vi "PC Streaming Host_2012.vi"() -> ()   [LabVIEW 2012]
uses:
  <vilib>/rvi/interface/nirviOpenFPGA/nirviOpenFPGA.xnode
  <vilib>/rvi/interface/nirviMethod/nirviMethod.xnode
  <vilib>/rvi/errors/niLvFpgaMergeErrorWithErrorCode.vi
  <vilib>/ptbypt/NI_PtbyPt.lvlib
  <vilib>/rvi/interface/nirviCloseFPGA/nirviCloseFPGA.xnode
  <vilib>/rvi/interface/nirviReadWriteControl/nirviReadWriteControl.xnode
  <vilib>/rvi/interface/Simulation/niFpgaSimulationCallBeginRW.vi
  <vilib>/rvi/errors/niLvFpgaAdjustHostInterfaceError.vi
  NiFpgaLv.dll
  <vilib>/Utility/error.llb/Error Cluster From Error Code.vi
  FPGA Bitfiles/TopLevelFPGA1.0.lvbitx
  Program Files/CAEN/HV/CAENHVWrapper/labview/CAENHVWrapper/CAENHVWrapper.lvlib
  <vilib>/FPGAPlugInAG/Dynamic/niLvFpga_ConfigureFifo_Dynamic.vi
  <vilib>/FPGAPlugInAG/Dynamic/niLvFpga_StartFifo_Dynamic.vi
  <vilib>/LabVIEW Targets/FPGA/FlexRIO/CustomFPGAMethods/79XXR_Method_IOModuleStatusImpl.vi
  <vilib>/FPGAPlugInAG/Dynamic/niLvFpga_Run_Dynamic.vi
  <vilib>/FPGAPlugInAG/Dynamic/niLvFpga_ReadFifo_Dynamic.vi
  <vilib>/FPGAPlugInAG/Dynamic/niLvFpga_Close_Dynamic.vi
  <vilib>/FPGAPlugInAG/PXI-7951R/niLvFpga_Open_PXI-7951R.vi
  <vilib>/rvi/interface/common/dynamic/niFpgaDynamicAddResources.vi
  <vilib>/userdefined/High Color/nirio_resource_hc.ctl
panel:
  out "Array":string[][](array[string])
  out "handle HV1":i32
  out "handle HV2":i32
  out "File name":string
  out "Total Data Chunks to Write":dbl
  in  "Tab Control":T1(tab)
  in  "Write mode":bool
  out "directory exists - please wait":u8(slide)
  out "directory ok":bool
  in  "Write Enable":bool=TRUE
  in  "File Path":path=path "C:/Users/admfroukjeg/Documents/test"
  in  "Number of Files to Write":u32=1
  in  "Save 10% of Data?":bool
  out "File Writing Progress (%)":dbl(slide) scale=0.0..100.0
  in  "Location":i16(ring)=1 items=["Purdue", "NIKHEF", "Zurich", "???"]
  in  "PXI address":T2="RIO0" caption="RIO Device"
  in  "Trigger level":i16[](array[numeric])=[4000, 4000, 4000, 4000, 4000, 4000, 4000, 4000] caption="Trigger"
  in  "Channel 0":bool=TRUE caption="Channel 1"
  in  "Channel 1":bool
  in  "Channel 2":bool caption="Channel 1"
  in  "Channel 3":bool caption="Channel 1"
  in  "Channel 4":bool caption="Channel 1"
  in  "Channel 5":bool caption="Channel 1"
  in  "Channel 6":bool caption="Channel 1"
  in  "Channel 7":bool caption="Channel 1"
  in  "Sources":string[](array[combo])
  in  "Serial numbers":string[](array[combo])
  in  "voltage":string[](array[string])=["100", "200", "300", "400", "500", "600", "700", "800"]
  in  "det_type":string[](array[combo])
  out "Voltage HV1":string[][](array[string])
  out "Voltage HV2":string[][](array[string])
  in  "IP adress HV1":string="1_0_0"
  in  "IP adress HV2":string="0_0_0"
  out "handle":i32
  in  "Master Pulser On/Off":bool
  in  "Pulse duration (samples)":u32
  in  "Pulse Separation (samples)":u32
  in  "Testpulse Turnaround Time (samples)":u32=14
  in  "circular buffer length (samples)":u32=1000
  in  "Pretrigger Samples":u32=15
  out "Samples per Data Chunk":u32
  in  "Waveforms per Data Chunk":u32=200 format="%.2p"
  in  "Samples per Waveform":u32=95
  in  "Data Chunks per File":u32=2
  out "Average Throughput":dbl(graph)
  out "Loop Time":u32
  out "Inst. Throughput":dbl format="%#_6p"
  out "Elements in FIFO":u32(graph)
  out "FIFO Overflow":bool
  out "Current Chunk":u32
  out "Current File":i32
  out "Trigger rate":dbl(graph)
  out "Waveform Graph":dynamicdata(graph)
  out "Channel number displayed":i16=-1
  out "XML String":string
  out "error out":errorcluster
  out "UTC format?":bool=TRUE
  out "Stopped":bool
  out "Channel On/Off":bool[](array[boolean])
  in  "stop 2":bool
  in  "stop":bool
  # "Only write every 10th chunk to disk"
  # "Program will stop when number of Files to Write is Complete OR if stop is pressed."
  # "Write continuously"
  # "Write finite number of files"
  # "TODO: Make this look like the \"detectors\" tab"
  # "Waveform/Data Chunk information"
  # "To compare directly on a scope: Horizontal scale: 200 ns/div Vertical scale: ~100 mV/div If 15 pretriggers, delay = 700 ns"
types:
  T1 = enum32{"File", "Detectors", "HV", "Pulser", "DAQ", "Host", "FIFO", "Trigger Rate", "Waveform Display", "XML", "Errors", "Misc."}
  T2 = typedef "nirio_resource_hc.ctl" = tag
  T3 = enum16{"open", "replace", "create", "open or create", "replace or create", "replace or create with confirmation"}
  T4 = enum16{"big-endian, network order", "native, host order", "little-endian"}
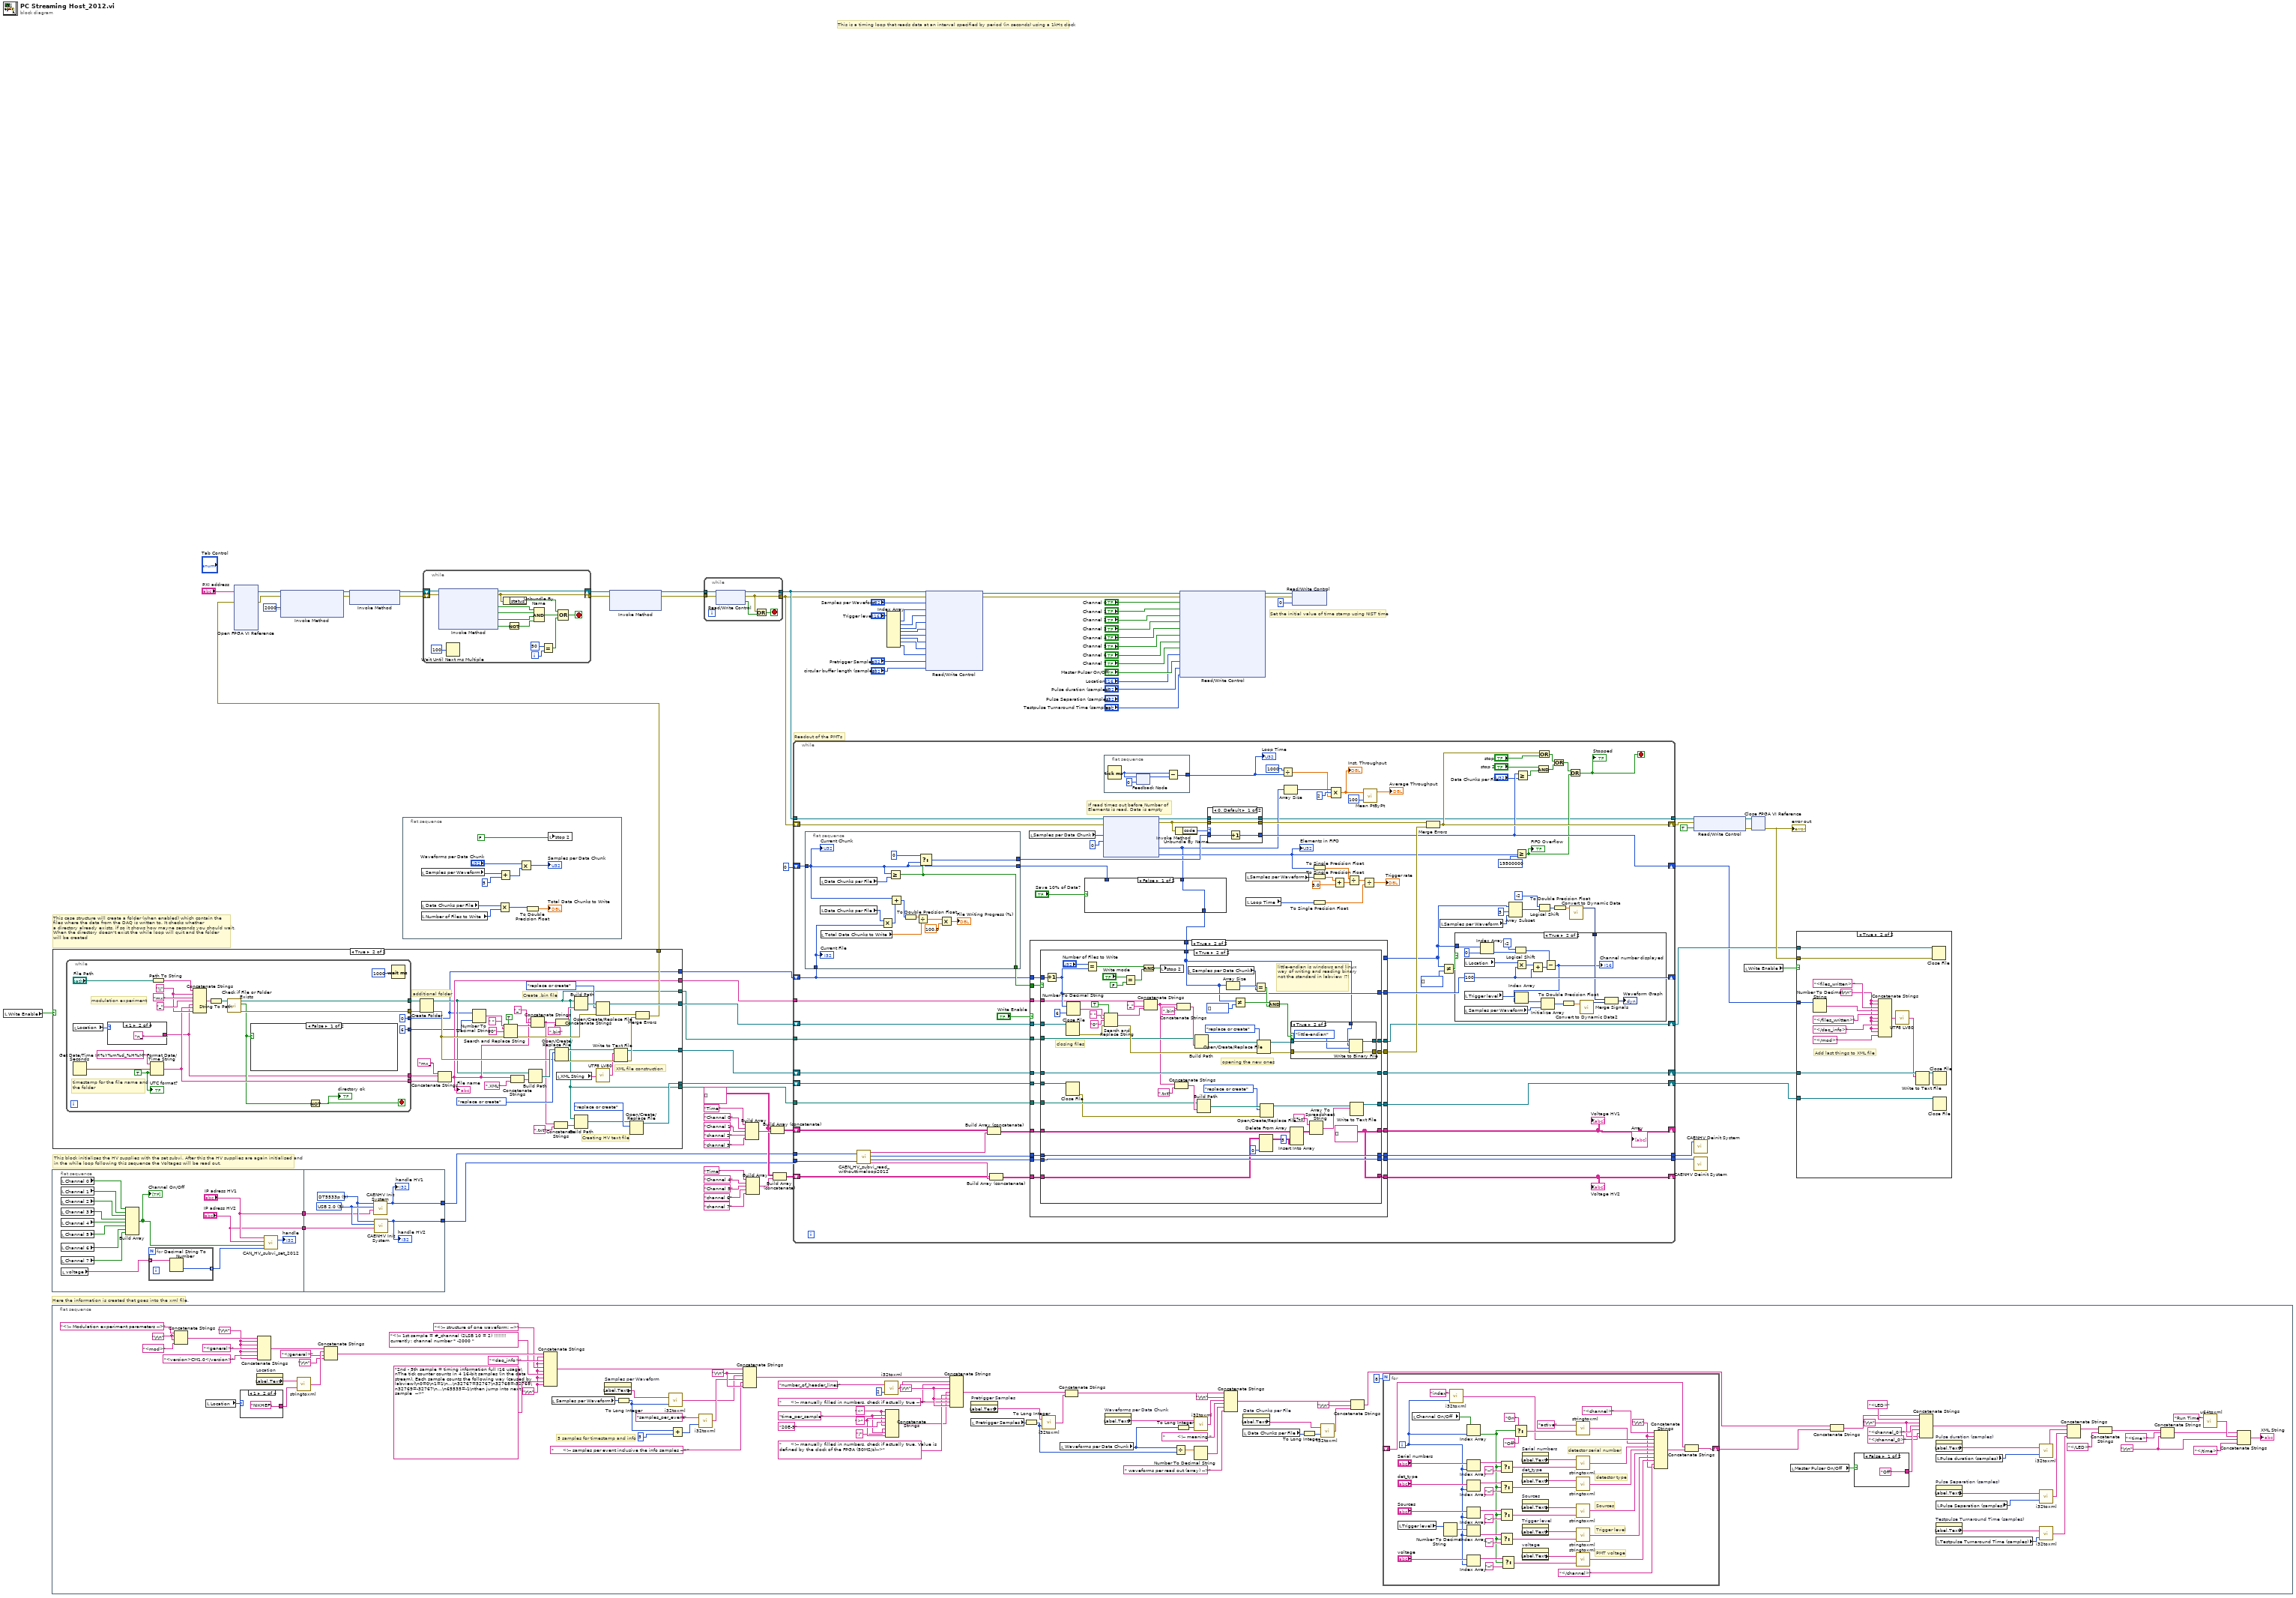
[diagram p0: block diagram]
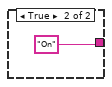
[diagram p2: hidden frame]
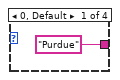
[diagram p3: hidden frame]
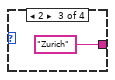
[diagram p4: hidden frame]
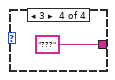
[diagram p5: hidden frame]
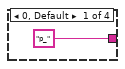
[diagram p7: hidden frame]
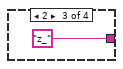
[diagram p8: hidden frame]
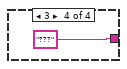
[diagram p9: hidden frame]
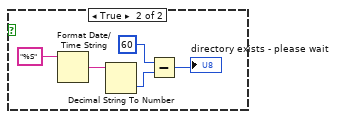
[diagram p10: hidden frame]
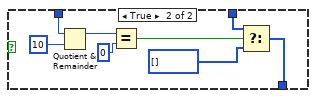
[diagram p13: hidden frame]
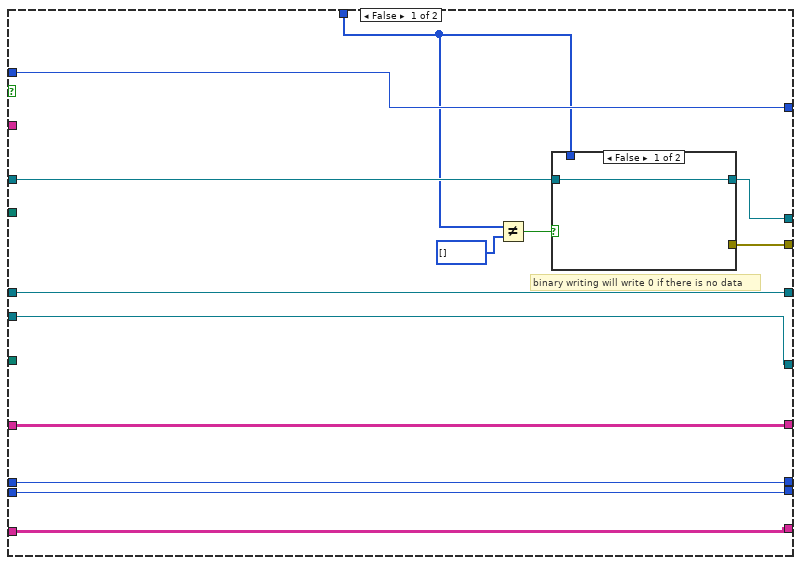
[diagram p15: hidden frame]
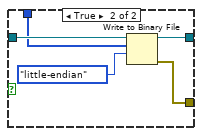
[diagram p16: hidden frame]
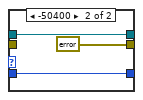
[diagram p18: hidden frame]
diagram:
  w9 = string[][] []
  # "Here the information is created that goes into the xml file."
  # "Readout of the PMTs"
  # "This block initialises the HV supplies with the set subvi. After this the HV supplies are again initialised and\nin the while loop following this sequence the Voltages will be read out."
  # "This case structure will create a folder (when enabled) which contain the \nfiles where the data from the DAQ is written to. It checks whether \na directory already exists, if so it shows how mayne seconds you should wait. \nWhen the directory doesn't exist the while loop will quit and the folder\nwill be created"
  # "This is a timing loop that reads data at an interval specified by period (in seconds) using a 1kHz clock"
  # "Set the initial value of time stamp using NIST time"
  n1 = local read "Write Enable"() -> (w77:bool)
  n2 = flat-sequence {
    frame #0 {
      w94 = "\r\n"
      w115 = "\r\n"
      w161 = ">" ("string")
      w158 = "<" ("string")
      w160 = "time_per_sample" ("variable name")
      w165 = "      <!-- manually filled in numbers, check if actually true -->" ("string")
      w166 = "\r\n"
      w175 = "\r\n"
      w121 = "\r\n"
      w129 = "\r\n"
      w179 = "\r\n"
      # "5 samples for timestamp and info"
      n3 = Concatenate Strings("<!-- Modulation experiment parameters -->", w179, w179, "<mod>" ("string")) -> (w132:string)
      n4 = local read "Location"() -> (w131:i16)
      n5 = case shown="1" w131 {
        tunnel: ["Purdue" "NIKHEF" "Zurich" "???"] -> w130
        frame 0, Default {
        }
        frame 1 {
        }
        frame 2 {
        }
        frame 3 {
        }
      }
      n6 = property on="Location" class="Ring (strict)"() -> ("Label.Text"=w106:string)  [unwired: 2 in, 2 out]
      n7 = Concatenate Strings(w132, w129, w129, "<general>" ("string"), w129, "<version>CM1.0</version>" ("string"), w129) -> (w133:string)
      n8 = call "stringtoxml.vi"("String to write"=w130, "XML Tag"=w106) -> ("xml string"=w128:string)
      n9 = Concatenate Strings(w133, w128, "</general>" ("string"), "\r\n") -> (w134:string)
      n10 = Concatenate Strings(w134, w121, "<daq_info>" ("string"), w121, "<!-- structure of one waveform: -->", w121, "<!-- 1st sample = #_channel (2LSB 10 = 2) !!!!!!!! currently: channel number * -2000 " ("string"), w121, "2nd - 5th sample = timing information full I16 usage\nThe tick counter counts in 4 16-bit samples (in the data stream). Each sample counts the following way (caused by labview)\n0=0\n1=1\n…\n32767=32767\n32768=-32768\n32769=-32767\n…\n65535=-1\nthen jump into next sample  -->" ("string"), w121) -> (w135:string)
      n11 = local read "Samples per Waveform"() -> (w167:u32)
      n12 = property on="Samples per Waveform" class="DigNum (strict)"() -> ("Label.Text"=w105:string)  [unwired: 2 in, 2 out]
      n13 = To Long Integer(number=w167) -> (32bit integer=w170:i32)
      n14 = call "i32toxml.vi"("variable"=w170, "variable name"=w105) -> ("xml string"=w168:string)
      n15 = Add(x=w170, y=5) -> (x+y=w172:i32)
      n16 = call "i32toxml.vi"("variable"=w172, "variable name"="samples_per_event") -> ("xml string"=w173:string)
      n17 = Concatenate Strings(w135, w175, w168, w173, "      <!-- samples per event inclusive the info samples -->" ("string"), w175) -> (w136:string)
      n18 = call "i32toxml.vi"("variable"=2, "variable name"="number_of_header_lines") -> ("xml string"=w155:string)
      n19 = Concatenate Strings(w158, w160, w161, "20E-9" ("string"), w158, "/" ("string"), w160, w161) -> (w163:string)
      n20 = Concatenate Strings(w136, w155, w165, w166, w163, "      <!-- manually filled in numbers, check if actually true. Value is defined by the clock of the FPGA (50MS/s)-->" ("string"), w166, w165, w166) -> (w137:string)
      n21 = property on="Pretrigger Samples" class="DigNum (strict)"() -> ("Label.Text"=w104:string)  [unwired: 2 in, 2 out]
      n22 = local read "Pretrigger Samples"() -> (w153:u32)
      n23 = To Long Integer(number=w153) -> (32bit integer=w144:i32)
      n24 = call "i32toxml.vi"("variable"=w144, "variable name"=w104) -> ("xml string"=w154:string)
      n25 = local read "Waveforms per Data Chunk"() -> (w149:u32)
      n26 = Concatenate Strings(w137, w154) -> (w138:string)
      n27 = property on="Waveforms per Data Chunk" class="DigNum (strict)"() -> ("Label.Text"=w103:string)  [unwired: 2 in, 2 out]
      n28 = Divide(x=w149, y=w144) -> (x/y=w148:dbl)
      n29 = To Long Integer(number=w149) -> (32bit integer=w147:i32)
      n30 = call "i32toxml.vi"("variable"=w147, "variable name"=w103) -> ("xml string"=w145:string)
      n31 = Number To Decimal String(number=w148) -> (decimal integer string=w151:string)  [unwired: 1 in]
      n32 = Concatenate Strings(w138, "\r\n", w145, "        <!-- meaning " ("string"), w151, " waveforms per read out (array) -->" ("string")) -> (w139:string)
      n33 = property on="Data Chunks per File" class="DigNum (strict)"() -> ("Label.Text"=w102:string)  [unwired: 2 in, 2 out]
      n34 = local read "Data Chunks per File"() -> (w142:u32)
      n35 = To Long Integer(number=w142) -> (32bit integer=w141:i32)
      n36 = call "i32toxml.vi"("variable"=w141, "variable name"=w102) -> ("xml string"=w140:string)
      n37 = Concatenate Strings(w139, "\r\n", w140) -> (w87:string)
      n38 = for {
        N: 8 -> [_]
        shift-right: [w184] -> w88
        shift-left: _ -> [w183]
        i -> [w191]
        w181 = "\r\n"
        # "PMT voltage"
        # "Trigger level"
        # "Sources"
        # "detector type"
        # "detector serial number"
        n39 = local read "Trigger level"() -> (w201:i16[])
        n40 = local read "Channel On/Off"() -> (w227:bool[])
        n41 = Number To Decimal String(number=w201) -> (decimal integer string=w198:string[])  [unwired: 1 in]
        n42 = call "i32toxml.vi"("variable"=w191, "variable name"="index") -> ("xml string"=w221:string)
        n43 = Index Array(array=w227, index=w191) -> (element=w190:bool)
        n44 = Index Array(array="Serial numbers", index=w191) -> (element=w218:string)
        n45 = Index Array(array="det_type", index=w191) -> (element=w211:string)
        n46 = Index Array(array="Sources", index=w191) -> (element=w206:string)
        n47 = Index Array(array=w198, index=w191) -> (element=w199:string)
        n48 = Index Array(array="voltage", index=w191) -> (element=w193:string)
        n49 = Select(t=w218, s=w190, f="--") -> (s? t:f=w216:string)
        n50 = Select(t=w211, s=w190, f="--") -> (s? t:f=w209:string)
        n51 = Select(t=w206, s=w190, f="--") -> (s? t:f=w203:string)
        n52 = Select(t=w199, s=w190, f="--") -> (s? t:f=w197:string)
        n53 = Select(t=w193, s=w190, f="--") -> (s? t:f=w189:string)
        n54 = Select(t="On" ("List Name"), s=w190, f="Off" ("List Name")) -> (s? t:f=w223:string)
        n55 = property on="Serial numbers" class="Arr (strict)"() -> ("Label.Text"=w215:string)  [unwired: 2 in, 2 out]
        n56 = property on="det_type" class="Arr (strict)"() -> ("Label.Text"=w210:string)  [unwired: 2 in, 2 out]
        n57 = property on="Sources" class="Arr (strict)"() -> ("Label.Text"=w204:string)  [unwired: 2 in, 2 out]
        n58 = property on="Trigger level" class="Arr (strict)"() -> ("Label.Text"=w196:string)  [unwired: 2 in, 2 out]
        n59 = property on="voltage" class="Arr (strict)"() -> ("Label.Text"=w188:string)  [unwired: 2 in, 2 out]
        n60 = call "stringtoxml.vi"("String to write"=w223, "XML Tag"="active") -> ("xml string"=w220:string)
        n61 = call "stringtoxml.vi"("String to write"=w216, "XML Tag"=w215) -> ("xml string"=w214:string)
        n62 = call "stringtoxml.vi"("String to write"=w209, "XML Tag"=w210) -> ("xml string"=w208:string)
        n63 = call "stringtoxml.vi"("String to write"=w203, "XML Tag"=w204) -> ("xml string"=w202:string)
        n64 = call "stringtoxml.vi"("String to write"=w197, "XML Tag"=w196) -> ("xml string"=w195:string)
        n65 = call "stringtoxml.vi"("String to write"=w189, "XML Tag"=w188) -> ("xml string"=w187:string)
        n66 = Concatenate Strings("<channel>" ("List Name"), w181, w221, w220, w214, w208, w202, w195, w187, "</channel>" ("List Name"), w181) -> (w185:string)
        n67 = Concatenate Strings(w183, w185) -> (w184:string)
      }
      n68 = local read "Master Pulser On/Off"() -> (w118:bool)
      n69 = Concatenate Strings(w87, w88) -> (w86:string)
      n70 = case shown="False" w118 {
        tunnel: ["Off" "On"] -> w117
        frame False {
        }
        frame True {
        }
      }
      n71 = Concatenate Strings(w86, "<LED>" ("string"), w115, "<channel_0>" ("string"), w117, "</channel_0>" ("string"), w115) -> (w113:string)
      n72 = property on="Pulse duration (samples)" class="DigNum (strict)"() -> ("Label.Text"=w101:string)  [unwired: 2 in, 2 out]
      n73 = local read "Pulse duration (samples)"() -> (w114:u32)
      n74 = property on="Pulse Separation (samples)" class="DigNum (strict)"() -> ("Label.Text"=w99:string)  [unwired: 2 in, 2 out]
      n75 = local read "Pulse Separation (samples)"() -> (w112:u32)
      n76 = property on="Testpulse Turnaround Time (samples)" class="DigNum (strict)"() -> ("Label.Text"=w100:string)  [unwired: 2 in, 2 out]
      n77 = local read "Testpulse Turnaround Time (samples)"() -> (w109:u32)
      n78 = call "i32toxml.vi"("variable"=w114, "variable name"=w101) -> ("xml string"=w111:string)
      n79 = call "i32toxml.vi"("variable"=w112, "variable name"=w99) -> ("xml string"=w110:string)
      n80 = call "i32toxml.vi"("variable"=w109, "variable name"=w100) -> ("xml string"=w108:string)
      n81 = Concatenate Strings(w113, w111, w110, w108) -> (w98:string)
      n82 = Concatenate Strings(w98, "</LED>" ("string")) -> (w97:string)
      n83 = Concatenate Strings(w97, "<time>" ("string"), w94) -> (w91:string)
      n84 = call "u64toxml.vi"("variable name"="Run Time") -> ("xml string"=w93:string)  [unwired: 1 in]
      n85 = Concatenate Strings(w91, w93, w94, "</time>" ("string")) -> (→"XML String":string)
    }
  }
  n86 = flat-sequence {
    tunnel: ["IP adress HV1"] -> w26
    tunnel: ["IP adress HV2"] -> w25
    tunnel: w26 -> [w253]
    tunnel: w25 -> [w252]
    tunnel: [w251] -> w4
    tunnel: [w250] -> w3
    frame #0 {
      n87 = local read "Channel 0"() -> (w243:bool)
      n88 = local read "Channel 1"() -> (w242:bool)
      n89 = local read "Channel 2"() -> (w241:bool)
      n90 = local read "Channel 3"() -> (w240:bool)
      n91 = local read "Channel 4"() -> (w239:bool)
      n92 = local read "Channel 5"() -> (w238:bool)
      n93 = local read "Channel 6"() -> (w237:bool)
      n94 = local read "Channel 7"() -> (w236:bool)
      n95 = local read "voltage"() -> (w234:string[])
      n96 = Build Array(w243, w242, w241, w240, w239, w238, w237, w236) -> (w235:bool[])
      "Channel On/Off" <- w235
      n97 = for {
        tunnel: w234 -> [w249] mode=indexing
        tunnel: [w248] -> w246 mode=indexing
        n98 = Decimal String To Number(string=w249) -> (number=w248:i32)  [unwired: 2 in, 1 out]
      }
      n99 = call "CAN_HV_subvi_set_2012.vi"("Voltage"=w246, "Power on/off"=w235, "IP adress HV2"="IP adress HV2", "IP adress HV1"="IP adress HV1") -> ("handle"=→"handle":i32)  [unwired: 1 out]
    }
    frame #1 {
      w255 = 3 items=["TCP/IP"=0, "HS CAENET"=2, "USB 2.0"=3, "CONET Optical Link"=4, "USB VCP"=5] ("LinkType")
      w254 = u32 9 items=["SY1527", "SY2527", "SY4527", "SY5527", "N568", "V65XX", "N1470", "V8100", "", "DT5533p"] ("system")
      n100 = call "CAENHV Init System.vi"("Arg"=w253, "LinkType"=w255, "system"=w254) -> ("handle"=w251:i32)  [unwired: 7 in, 1 out]
      "handle HV1" <- w251
      n101 = call "CAENHV Init System.vi"("Arg"=w252, "LinkType"=w255, "system"=w254) -> ("handle"=w250:i32)  [unwired: 7 in, 1 out]
      "handle HV2" <- w250
    }
  }
  n102 = case shown="True" w77 {
    tunnel: [_ w287] -> w76
    tunnel: [_ w268] -> w31
    tunnel: [_ w258] -> w8
    tunnel: [_ w265] -> w29
    tunnel: [_ w266] -> w28
    tunnel: [_ w259] -> w5
    tunnel: [_ w258] -> w6
    tunnel: [_ w256] -> w2
    frame False {
    }
    frame True {
      # "Create .bin file"
      # "Creating HV text file"
      # "XML file construction"
      # "additional folder"
      n103 = while {
        tunnel: [w306] -> w267
        tunnel: [w304] -> w272
        tunnel: [w303] -> w271
        tunnel: [w298] -> w270
        tunnel: [0 ("number")] -> w256
        tunnel: [i16 6 ("width (-)")] -> w257
        stop <- w300 stop-if-true
        w307 = "\\" ("string")
        w309 = TRUE ("UTC format")
        # "modulation experiment"
        # "timestamp for the file name and the folder"
        n104 = local read "Location"() -> (w299:i16)
        n105 = Get Date/Time In Seconds() -> (seconds since 1Jan1904=w310:timestamp)
        n106 = case shown="1" w299 {
          tunnel: ["p_" ("string") "n_" ("string") "z_" ("string") "???"] -> w298
          frame 0, Default {
          }
          frame 1 {
          }
          frame 2 {
          }
          frame 3 {
          }
        }
        n107 = Format Date/Time String(time format string (%c)="%Y%m%d_%H%M", seconds (now)=w310, UTC format=w309) -> (date/time string=w306:string)
        n108 = Path To String(path="File Path") -> (string=w312:string)
        n109 = Concatenate Strings(w312, w307, "mx" ("string"), "_" ("string"), w298, w306, w307) -> (w315:string)
        n110 = String To Path(string=w315) -> (path=w305:path)
        n111 = call <vilib>:"Check if File or Folder Exists.vi"("path"=w305) -> ("error out"=w304:errorcluster, "file or folder exists?"=w302:bool, "dup path"=w303:path)  [unwired: 8 in]
        n112 = case shown="False" w302 {
          frame False {
          }
          frame True {
            n113 = Format Date/Time String(time format string (%c)="%S") -> (date/time string=w323:string)  [unwired: 2 in]
            n114 = Decimal String To Number(string=w323) -> (number=w321:i32)  [unwired: 2 in, 1 out]
            n115 = Subtract(x=60, y=w321) -> (x-y=→"directory exists - please wait":i32)
          }
        }
        n116 = Not(x=w302) -> (.not. x?=w300:bool)
        "directory ok" <- w300
        n117 = Wait (ms)(milliseconds to wait=1000) -> ()  [unwired: 1 out]
        "UTC format?" <- w309
      }
      n118 = Create Folder(path (use dialog)=w271, error in=w272) -> (created path=w258:path, error out=w283:errorcluster)  [unwired: 1 in, 1 out]
      n119 = Concatenate Strings("mx_" ("string"), w270, w267) -> (w265:string)
      "File name" <- w265
      n120 = Number To Decimal String(number=w256, width (-)=w257) -> (decimal integer string=w294:string)
      n121 = Search and Replace String(replace all?=TRUE ("replace all? (F)"), input string=w294, search string=" ", replace string="0" ("replace string (\"\")"), error in=w283) -> (result string=w275:string, error out=w289:errorcluster)  [unwired: 3 in, 2 out]
      n122 = Concatenate Strings(w265, ".XML" ("substring (\"\")")) -> (w280:string)
      n123 = Build Path(base path=w258, name or relative path=w280) -> (appended path=w285:path)
      n124 = Concatenate Strings(w265, "_" ("string"), w275) -> (w261:string)
      n125 = Concatenate Strings(w261, ".txt" ("string")) -> (w262:string)
      n126 = Open/Create/Replace File(file path (use dialog)=w285, error in=w283, operation (0:open)=T3."replace or create") -> (refnum out=w276:refnum<file>, error out=w278:errorcluster)  [unwired: 3 in, 1 out]
      n127 = Concatenate Strings(w261, ".bin" ("substring (\"\")")) -> (w282:string)
      n128 = local read "XML String"() -> (w273:string)
      n129 = Build Path(base path=w258, name or relative path=w282) -> (appended path=w290:path)
      n130 = Build Path(base path=w258, name or relative path=w262) -> (appended path=w263:path)
      n131 = call "UTF8 LV80.vi"("text"=w273) -> ("utf-8 text out"=w274:string)
      n132 = Open/Create/Replace File(file path (use dialog)=w290, error in=w289, operation (0:open)=T3."replace or create") -> (refnum out=w287:refnum<file>, error out=w286:errorcluster)  [unwired: 3 in, 1 out]
      n133 = Write to Text File(file (use dialog)=w276, text=w274, error in=w278) -> (refnum out=w268:refnum<file>, error out=w277:errorcluster)  [unwired: 1 in, 1 out]
      n134 = Open/Create/Replace File(file path (use dialog)=w263, operation (0:open)=T3."replace or create") -> (refnum out=w259:refnum<file>)  [unwired: 4 in, 2 out]
      n135 = Merge Errors(w286, w277) -> (w266:errorcluster)
    }
  }
  n136 = xnode "Open FPGA VI Reference"("error in"=w28, "resource name"="PXI address") -> ("FPGA VI Reference Out"=w85:refnum<k20>, "error out"=w84:errorcluster)
  n137 = xnode "Invoke Method"("FPGA VI Reference In"=w85, "error in"=w84, "Requested Depth"=u32 20000000) -> ("FPGA VI Reference Out"=w56:refnum<k20>, "error out"=w55:errorcluster)  [unwired: 1 out]
  n138 = xnode "Invoke Method"("FPGA VI Reference In"=w56, "error in"=w55) -> ("FPGA VI Reference Out"=w43:refnum<k20>, "error out"=w42:errorcluster)
  n139 = flat-sequence {
    frame #0 {
      n140 = local read "Samples per Waveform"() -> (w332:u32)
      n141 = local read "Data Chunks per File"() -> (w329:u32)
      n142 = local read "Number of Files to Write"() -> (w328:u32)
      n143 = Multiply(x=w329, y=w328) -> (x*y=w327:u32)
      n144 = Add(x=w332, y=u32 5) -> (x+y=w334:u32)
      n145 = Multiply(x="Waveforms per Data Chunk", y=w334) -> (x*y=→"Samples per Data Chunk":u32)
      n146 = To Double Precision Float(number=w327) -> (double precision float=→"Total Data Chunks to Write":dbl)
      n147 = local write "stop 2"(FALSE ("stop 2")) -> ()
    }
  }
  n148 = while {
    shift-right: [w341] -> w81
    shift-left: w42 -> [w349]
    shift-right: [w348] -> w47
    shift-left: w43 -> [w350]
    i -> [w343]
    stop <- w338 stop-if-true
    n149 = xnode "Invoke Method"("FPGA VI Reference In"=w350, "error in"=w349) -> ("FPGA VI Reference Out"=w348:refnum<k20>, "error out"=w341:errorcluster, "IO Module Present?"=w347:bool, "Power Enabled?"=w346:bool, "IO Enabled?"=w345:bool, "IO Module Mismatch?"=w336:bool)
    n150 = Wait Until Next ms Multiple(millisecond multiple=u32 100) -> ()  [unwired: 1 out]
    n151 = Unbundle By Name(w341) -> ("status"=w340:bool)
    n152 = Not(x=w336) -> (.not. x?=w335:bool)
    n153 = Compound Arithmetic op=AND(w347, w346, w345, w335) -> (w339:bool)
    n154 = Equal?(x=50, y=w343) -> (x = y?=w337:bool)
    n155 = Compound Arithmetic op=OR(w340, w339, w337) -> (w338:bool)
  }
  n156 = xnode "Invoke Method"("FPGA VI Reference In"=w47, "error in"=w81) -> ("FPGA VI Reference Out"=w82:refnum<k20>, "error out"=w83:errorcluster)  [unwired: 1 in]
  n157 = while {
    tunnel: [w351] -> w30
    tunnel: [w356] -> w46
    tunnel: w82 -> [w355]
    tunnel: w83 -> [w354]
    stop <- w352 stop-if-true
    n158 = xnode "Read/Write Control"("FPGA VI Reference In"=w355, "error in"=w354) -> ("FPGA VI Reference Out"=w356:refnum<k20>, "error out"=w351:errorcluster, "Init Done"=w353:bool)
    n159 = Or(x=w351, y=w353) -> (x .or. y?=w352:bool)
  }
  n160 = Build Array("Time", "Channel 0", "Channel 1", "channel 2", "channel 3") -> (w18:string[])
  n161 = Build Array("Time", "Channel 4", "Channel 5", "channel 6", "channel 7") -> (w10:string[])
  n162 = Build Array (concatenate)(w9, w18) -> (w17:string[][])
  n163 = Build Array (concatenate)(w9, w10) -> (w11:string[][])
  n164 = while {
    shift-right: [w422] -> w48
    shift-left: w30 -> [w394]
    tunnel: w29 -> [w427]
    shift-right: [w413] -> w61
    shift-left: u32 0 -> [w378]
    tunnel: w8 -> [w428]
    shift-right: [w424] -> _
    shift-left: w2 -> [w396]
    shift-right: [w419] -> w75
    shift-left: w76 -> [w420]
    shift-right: [w416] -> w74
    shift-left: w31 -> [w417]
    tunnel: w46 -> [w395]
    tunnel: [w374] -> w49
    shift-right: [w359] -> _
    shift-left: w17 -> [w371]
    shift-right: [w358] -> _
    shift-left: w11 -> [w370]
    tunnel: w3 -> [w369]
    tunnel: [w363] -> w24
    shift-right: [w368] -> w7
    shift-left: w5 -> [w366]
    tunnel: w6 -> [w367]
    tunnel: w4 -> [w365]
    tunnel: [w362] -> w1
    stop <- w379 stop-if-true
    # "If read times out before Number of Elements is read, Data is empty"
    n165 = flat-sequence {
      tunnel: [w452] -> w426
      tunnel: [w451] -> w425
      tunnel: w396 -> [w449]
      tunnel: w378 -> [w440]
      tunnel: [w440] -> w377
      frame #0 {
        n166 = local read "Data Chunks per File"() -> (w450:u32)
        n167 = local read "Data Chunks per File"() -> (w448:u32)
        n168 = local read "Total Data Chunks to Write"() -> (w444:dbl)
        n169 = Multiply(x=w448, y=w449) -> (x*y=w447:u32)
        n170 = Greater Or Equal?(x=w440, y=w450) -> (x >= y?=w451:bool)
        n171 = Add(x=w440, y=w447) -> (x+y=w446:u32)
        n172 = To Double Precision Float(number=w446) -> (double precision float=w445:dbl)
        n173 = Divide(x=w445, y=w444) -> (x/y=w442:dbl)
        n174 = Select(t=u32 0, s=w451, f=w440) -> (s? t:f=w452:u32)
        n175 = Multiply(x=w442, y=100.0) -> (x*y=→"File Writing Progress (%)":dbl)
        "Current Chunk" <- w440
        "Current File" <- w449
      }
    }
    n176 = call "CAEN_HV_subvi_read_withouttimeloop2012.vi"("handle HV1"=w365, "handle HV2"=w369) -> ("Time&Voltage HV1"=w372:string[], "handle HV1 out"=w361:i32, "handle HV2 out"=w364:i32, "Time&Voltage HV2"=w373:string[])
    n177 = Build Array (concatenate)(w371, w372) -> (w360:string[][])
    n178 = Build Array (concatenate)(w370, w373) -> (w357:string[][])
    n179 = local read "Samples per Data Chunk"() -> (w397:u32)
    n180 = xnode "Invoke Method"("FPGA VI Reference In"=w395, "error in"=w394, "Number of Elements"=w397, "Timeout (ms)"=0) -> ("FPGA VI Reference Out"=w375:refnum<k20>, "error out"=w437:errorcluster, "Data"=w376:i16[], "Elements Remaining"=w393:u32)
    "Elements in FIFO" <- w393
    n181 = case shown="False" "Save 10% of Data?" {
      tunnel: [w472 w475] -> w401
      tunnel: w376 -> [w472 w474]
      tunnel: w377 -> [_ w473]
      frame False {
      }
      frame True {
        n182 = Quotient & Remainder(x=w473, y=u32 10) -> (x-y*floor(x/y)=w479:u32)  [unwired: 1 out]
        n183 = Equal?(x=w479, y=u32 0) -> (x = y?=w477:bool)
        n184 = Select(t=w474, s=w477, f=i16[] [] ("y")) -> (s? t:f=w475:i16[])
      }
    }
    n185 = case shown="True" "Write Enable" {
      tunnel: w401 -> [w491 w508]
      tunnel: [w491 _] -> w398
      tunnel: w428 -> [_ w515]
      tunnel: w427 -> [_ w505]
      tunnel: w425 -> [_ w514]
      tunnel: w396 -> [w493 w513]
      tunnel: [w493 w512] -> w424
      tunnel: [_ w511] -> w421
      tunnel: [w492 w510] -> w419
      tunnel: w420 -> [w492 w509]
      tunnel: w417 -> [w490 w507]
      tunnel: [w490 w506] -> w416
      tunnel: w366 -> [w489 w504]
      tunnel: w367 -> [_ w503]
      tunnel: [w489 w502] -> w368
      tunnel: w364 -> [w487 w501]
      tunnel: [w487 w500] -> w363
      tunnel: [w488 w499] -> w362
      tunnel: w361 -> [w488 w498]
      tunnel: w360 -> [w486 w497]
      tunnel: [w486 w496] -> w359
      tunnel: [w485 w494] -> w358
      tunnel: w357 -> [w485 w495]
      frame False {
      }
      frame True {
        n186 = case shown="True" w514 {
          tunnel: w515 -> [_ w571]
          tunnel: w508 -> [w522 w556]
          tunnel: [w521 w570] -> w511
          tunnel: w509 -> [w527 w584]
          tunnel: w513 -> [w528 w585]
          tunnel: [w528 w563] -> w512
          tunnel: [w526 w577] -> w510
          tunnel: w507 -> [w525 w572]
          tunnel: [w525 w572] -> w506
          tunnel: w505 -> [_ w557]
          tunnel: w504 -> [w520 w555]
          tunnel: w503 -> [_ w551]
          tunnel: [w520 w536] -> w502
          tunnel: w501 -> [w518 w547]
          tunnel: [w518 w547] -> w500
          tunnel: [w519 w546] -> w499
          tunnel: w498 -> [w519 w546]
          tunnel: [w517 w535] -> w496
          tunnel: w497 -> [w517 w542]
          tunnel: w495 -> [w516 w544]
          tunnel: [w516 w535] -> w494
          frame False {
            # "binary writing will write 0 if there is no data"
            n187 = Not Equal?(x=w522, y=i16[] []) -> (x != y?=w523:bool)
            n188 = case shown="False" w523 {
              tunnel: w527 -> [w529 w534]
              tunnel: [w529 w533] -> w526
              tunnel: [_ w532] -> w521
              tunnel: w522 -> [_ w530]
              frame False {
              }
              frame True {
                n189 = Write to Binary File(file (use dialog)=w534, data=w530, 9:T4."little-endian" ("byte order (0:big-endian, network order)")) -> (refnum out=w533:refnum<file>, error out=w532:errorcluster)  [unwired: 3 in, 1 out]
              }
            }
          }
          frame True {
            w535 = string[][] []
            # "opening the new ones"
            # "closing files"
            # "little-endian is windows and linux way of writing and reading binary not the standard in labview !?!"
            n190 = Increment(x=w585) -> (x+1=w563:i32)
            n191 = Close File(refnum=w584) -> (error out=w583:errorcluster)  [unwired: 1 in, 1 out]
            n192 = Close File(refnum=w555) -> (error out=w548:errorcluster)  [unwired: 1 in, 1 out]
            n193 = Number To Decimal String(number=w563, width (-)=i16 6) -> (decimal integer string=w587:string)
            n194 = Equal?(x="Number of Files to Write", y=w563) -> (x = y?=w558:bool)
            n195 = Search and Replace String(replace all?=TRUE ("replace all? (F)"), input string=w587, search string=" ", replace string="0" ("replace string (\"\")"), error in=w583) -> (result string=w576:string, error out=w582:errorcluster)  [unwired: 3 in, 2 out]
            n196 = Equal?(x="Write mode", y=FALSE) -> (x = y?=w559:bool)
            n197 = And(x=w558, y=w559) -> (x .and. y?=w560:bool)
            n198 = Concatenate Strings(w557, "_" ("string"), w576) -> (w554:string)
            n199 = local write "stop 2"(w560) -> ()
            n200 = Concatenate Strings(w554, ".txt" ("string")) -> (w552:string)
            n201 = Concatenate Strings(w554, ".bin" ("substring (\"\")")) -> (w574:string)
            n202 = local read "Samples per Data Chunk"() -> (w567:u32)
            n203 = Build Path(base path=w571, name or relative path=w574) -> (appended path=w581:path)
            n204 = Build Path(base path=w551, name or relative path=w552) -> (appended path=w550:path)
            n205 = Array Size(array=w556) -> (size(s)=w568:i32)
            n206 = Not Equal?(x=w556, y=i16[] []) -> (x != y?=w569:bool)
            n207 = Equal?(x=w568, y=w567) -> (x = y?=w566:bool)
            n208 = Open/Create/Replace File(file path (use dialog)=w581, error in=w582, operation (0:open)=T3."replace or create") -> (refnum out=w578:refnum<file>, error out=w579:errorcluster)  [unwired: 3 in, 1 out]
            n209 = Delete From Array(array=w544, index (col)=0 ("disabled index (col)")) -> (array with subset deleted=w541:string[][])  [unwired: 2 in, 1 out]
            n210 = Open/Create/Replace File(file path (use dialog)=w550, error in=w548, operation (0:open)=T3."replace or create") -> (refnum out=w545:refnum<file>)  [unwired: 3 in, 2 out]
            n211 = And(x=w569, y=w566) -> (x .and. y?=w565:bool)
            n212 = Insert Into Array(array=w542, index (col)=5 ("disabled index (col)"), new element=w541) -> (w539:string[][])  [unwired: 1 in]
            n213 = case shown="True" w565 {
              tunnel: w579 -> [w592 w599]
              tunnel: w578 -> [w593 w598]
              tunnel: [w593 w597] -> w577
              tunnel: [w592 w596] -> w570
              tunnel: w556 -> [_ w595]
              frame False {
              }
              frame True {
                n214 = Write to Binary File(file (use dialog)=w598, data=w595, error in=w599, 9:T4."little-endian" ("byte order (0:big-endian, network order)")) -> (refnum out=w597:refnum<file>, error out=w596:errorcluster)  [unwired: 2 in, 1 out]
              }
            }
            n215 = Array To Spreadsheet String(array=w539, 3:"%s" ("format string")) -> (spreadsheet string=w537:string)  [unwired: 1 in]
            n216 = Write to Text File(file (use dialog)=w545, text=w537) -> (refnum out=w536:refnum<file>)  [unwired: 2 in, 2 out]
          }
        }
      }
    }
    "Voltage HV2" <- w358
    "Voltage HV1" <- w359
    "Array" <- w359
    n217 = flat-sequence {
      tunnel: [w484] -> w431
      frame #0 {
        n218 = Tick Count (ms)() -> (millisecond timer value=w483:u32)
        n219 = feedback #1(u32 0 ("millisecond timer value")) -> (w482:u32)
        n220 = feedback-in #1(w483) -> ()
        n221 = Subtract(x=w483, y=w482) -> (x-y=w484:u32)
      }
    }
    n222 = Unbundle By Name(w437) -> ("code"=w438:i32)
    n223 = case shown="0, Default" w438 {
      tunnel: [w603 errorcluster {"status"=FALSE, "code"=0, "source"=""} ("error constant")] -> w423
      tunnel: w437 -> [w603 _]
      tunnel: w426 -> [w602 w605]
      tunnel: [w601 w605] -> w413
      tunnel: [w600 w604] -> w374
      tunnel: w375 -> [w600 w604]
      frame 0, Default {
        n224 = Increment(x=w602) -> (x+1=w601:u32)
      }
      frame -50400 {
      }
    }
    n225 = local read "Samples per Waveform"() -> (w389:u32)
    n226 = local read "Loop Time"() -> (w386:u32)
    n227 = Divide(x=u32 1000, y=w431) -> (x/y=w433:dbl)
    n228 = Array Size(array=w376) -> (size(s)=w436:i32)
    n229 = To Single Precision Float(number=w393) -> (single precision float=w392:sgl)
    n230 = To Single Precision Float(number=w389) -> (single precision float=w388:sgl)
    n231 = To Single Precision Float(number=w386) -> (single precision float=w385:sgl)
    n232 = Compound Arithmetic op=MULTIPLY(w436, 2 ("y"), w433) -> (w430:dbl)
    "Inst. Throughput" <- w430
    n233 = Add(x=w388, y=5.0) -> (x+y=w391:dbl)
    n234 = Divide(x=w392, y=w391) -> (x/y=w387:dbl)
    n235 = Divide(x=w387, y=w385) -> (x/y=→"Trigger rate":dbl)
    n236 = call <vilib>:"Mean PtByPt.vi"("x"=w430, "sample length"=100) -> ("mean"=→"Average Throughput":dbl)  [unwired: 2 in, 1 out]
    n237 = Merge Errors(w423, w421) -> (w422:errorcluster)
    n238 = local read "Samples per Waveform"() -> (w406:u32)
    n239 = Not Equal?(x=w398, y=i16[] []) -> (x != y?=w399:bool)
    n240 = Array Subset(array=w398, index=5, length=w406) -> (w381:i16[])
    n241 = Greater Or Equal?(x=w393, y=u32 19500000) -> (x >= y?=w404:bool)
    "FIFO Overflow" <- w404
    n242 = Greater Or Equal?(x=w413, y="Data Chunks per File") -> (x >= y?=w415:bool)
    n243 = And(x="stop 2", y=w415) -> (x .and. y?=w414:bool)
    n244 = Or(x=w422, y="stop") -> (x .or. y?=w411:bool)
    n245 = Logical Shift(y=i16 -2, x=w381) -> (x << y=w380:i16[])
    n246 = Or(x=w411, y=w414) -> (x .or. y?=w409:bool)
    n247 = To Double Precision Float(number=w380) -> (double precision float=w405:dbl[])
    n248 = Or(x=w409, y=w404) -> (x .or. y?=w379:bool)
    "Stopped" <- w379
    n249 = call "Convert to Dynamic Data"("Array"=w405) -> ("Dynamic Data Type"=w383:dynamicdata)  [unwired: 3 in]
    n250 = case shown="True" w399 {
      tunnel: w398 -> [_ w470]
      tunnel: w383 -> [_ w457]
      frame False {
      }
      frame True {
        w464 = i16 100
        n251 = local read "Location"() -> (w463:i16)
        n252 = local read "Trigger level"() -> (w459:i16[])
        n253 = local read "Samples per Waveform"() -> (w461:u32)
        n254 = Index Array(array=w470, index=0) -> (element=w467:i16)
        n255 = Logical Shift(y=i16 -2, x=w467) -> (x << y=w469:i16)
        n256 = Multiply(x=w463, y=w464) -> (x*y=w465:i16)
        n257 = Add(x=w465, y=w464) -> (x+y=w466:i16)
        n258 = Subtract(x=w469, y=w466) -> (x-y=w454:i16)
        "Channel number displayed" <- w454
        n259 = Index Array(array=w459, index=w454) -> (element=w460:i16)
        n260 = Initialize Array(w460, w461) -> (w455:i16[])
        n261 = To Double Precision Float(number=w455) -> (double precision float=w462:dbl[])
        n262 = call "Convert to Dynamic Data2"("Array"=w462) -> ("Dynamic Data Type"=w456:dynamicdata)  [unwired: 3 in]
        n263 = Merge Signals(w457, w456) -> (→"Waveform Graph":dynamicdata)
      }
    }
    "Loop Time" <- w431
  }
  n264 = Index Array(array="Trigger level") -> (element #1=w39:i16, element #2=w38:i16, element #3=w37:i16, element #4=w36:i16, element #5=w35:i16, element #6=w34:i16, element #7=w32:i16, element #8=w33:i16)  [unwired: 8 in]
  n265 = xnode "Read/Write Control"("FPGA VI Reference In"=w46, "error in"=w30, "Record Size only data"="Samples per Waveform", "Trigger 0"=w39, "Trigger 1"=w38, "Trigger 2"=w37, "Trigger 3"=w36, "Trigger 4"=w35, "Trigger 5"=w34, "Trigger 6"=w32, "Trigger 7"=w33, "# of pretrigger"="Pretrigger Samples", "circular buffer length"="circular buffer length (samples)") -> ("FPGA VI Reference Out"=w70:refnum<k20>, "error out"=w69:errorcluster)
  n266 = xnode "Read/Write Control"("FPGA VI Reference In"=w70, "error in"=w69, "channel 0 on/off"="Channel 0", "channel 1 on/off"="Channel 1", "channel 2 on/off"="Channel 2", "channel 3 on/off"="Channel 3", "channel 4 on/off"="Channel 4", "channel 5 on/off"="Channel 5", "channel 6 on/off"="Channel 6", "channel 7 on/off"="Channel 7", "location"="Location", "Testpulser On/Off"="Master Pulser On/Off", "Testpulse duration (20 ns ticks)"="Pulse duration (samples)", "Testpulse Time Delay (20 ns ticks)"="Testpulse Turnaround Time (samples)") -> ("FPGA VI Reference Out"=w45:refnum<k20>, "error out"=w44:errorcluster)
  n267 = xnode "Read/Write Control"("FPGA VI Reference In"=w45, "error in"=w44, "initial value"=u64 0) -> ()  [unwired: 2 out]
  n268 = xnode "Read/Write Control"("FPGA VI Reference In"=w49, "error in"=w48, "Stop FPGA and exit"=TRUE) -> ("FPGA VI Reference Out"=w54:refnum<k20>, "error out"=w53:errorcluster)
  n269 = call "CAENHV Deinit System.vi"("handle"=w1) -> ()  [unwired: 10 in, 1 out]
  n270 = call "CAENHV Deinit System.vi"("handle"=w24) -> ()  [unwired: 10 in, 1 out]
  n271 = local read "Write Enable"() -> (w78:bool)
  n272 = xnode "Close FPGA VI Reference"("FPGA VI Reference In"=w54, "error in"=w53) -> ("error out"=w79:errorcluster)
  "error out" <- w79
  n273 = case shown="True" w78 {
    tunnel: w79 -> [_ w611]
    tunnel: w75 -> [_ w620]
    tunnel: w74 -> [_ w619]
    tunnel: w61 -> [_ w614]
    tunnel: w7 -> [_ w607]
    frame False {
    }
    frame True {
      w608 = "\r\n"
      # "Add last things to XML file"
      n274 = Number To Decimal String(number=w614) -> (decimal integer string=w616:string)  [unwired: 1 in]
      n275 = Concatenate Strings(w608, w608, "<files_written> " ("text"), w616, "</files_written>" ("string"), w608, w608, "</daq_info>" ("string"), w608, w608, "</mod>" ("string")) -> (w610:string)
      n276 = call "UTF8 LV80.vi"("text"=w610) -> ("utf-8 text out"=w612:string)
      n277 = Write to Text File(file (use dialog)=w619, text=w612) -> (refnum out=w618:refnum<file>)  [unwired: 2 in, 2 out]
      n278 = Close File(refnum=w620, error in=w611) -> ()  [unwired: 2 out]
      n279 = Close File(refnum=w618) -> ()  [unwired: 1 in, 2 out]
      n280 = Close File(refnum=w607) -> ()  [unwired: 1 in, 2 out]
    }
  }
